vi "Process Image.vi"(4 "Path Angle":dbl, 6 "Camera Angle":dbl, 7 "?":T1, 8 "Error In":errorcluster, 9 "FOV":dbl[](array[numeric]), 10 "Process Memory":T2, 11 "Acquired Image":T2) -> (0 "Error Out":errorcluster, 1 "Particle Locations":dbl[][](array[numeric]) format="%.2f", 3 "Processed Image":T2)   [LabVIEW 2018]
uses:
  <vilib>/vision/Image Controls.llb/IMAQ Image.ctl
  <vilib>/vision/NI_Vision_Development_Module.lvlib
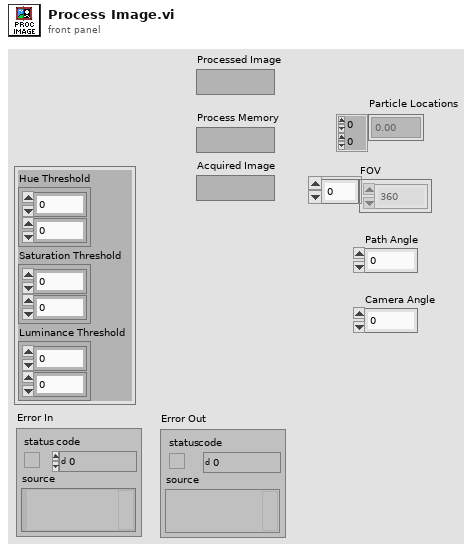
[diagram p1: front panel]
types:
  T1 = cluster{"Hue Threshold":cluster{i32, i32}, "Saturation Threshold":cluster{i32, i32}, "Luminance Threshold":cluster{i32, i32}}
  T2 = typedef "IMAQ Image.ctl" = refnum<image>
  T3 = cluster{"Blue or Luma":u8, "Green or Sat Plane":u8, "Red or Hue Plane":u8, "Alpha":u8}
  T4 = typedef "IMAQ Circle" = cluster{"Center X":i32, "Center Y":i32, "Inner Radius":i32, "Outer Radius":i32, "Start Angle":dbl, "End Angle":dbl}
  T5 = typedef "Particle Parameters" = i32
  T6 = typedef "ROI Descriptor" = cluster{"Global Rectangle":i32[], "Contours":cluster{"ID":enum32{"External", "Internal"}, "Type":u32, "Coordinates":i32[]}[]}
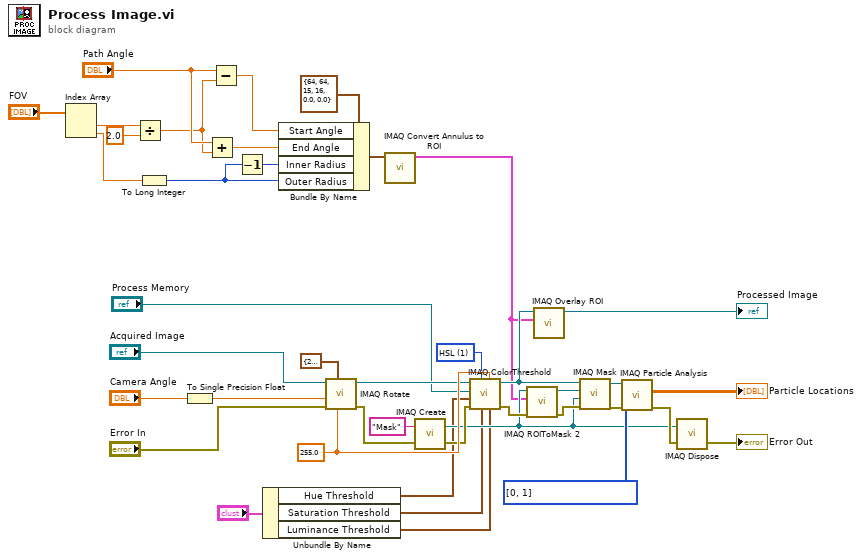
[diagram p0: block diagram]
diagram:
  w2 = u16 1 items=["RGB", "HSL", "HSV", "HSI"] ("Color Mode")
  w34 = T5[] [0, 1] items=["Center of Mass X", "Center of Mass Y", "First Pixel X", "First Pixel Y", "Bounding Rect Left", "Bounding Rect Top", "Bounding Rect Right", "Bounding Rect Bottom", "Max Feret Diameter Start X", "Max Feret Diameter Start Y", "Max Feret Diameter End X", "Max Feret Diameter End Y", "Max Horiz. Segment Length Left", "Max Horiz. Segment Length Right", "Max Horiz. Segment Length Row", "-", "Bounding Rect Width", "Bounding Rect Height", "Bounding Rect Diagonal", "Perimeter", "Convex Hull Perimeter", "Holes' Perimeter", "Max Feret Diameter", "Equivalent Ellipse Major Axis", "Equivalent Ellipse Minor Axis", "Equivalent Ellipse Minor Axis (Feret)", "Equivalent Rect Long Side", "Equivalent Rect Short Side", "Equivalent Rect Diagonal", "Equivalent Rect Short Side (Feret)", "Average Horiz. Segment Length", "Average Vert. Segment Length", "Hydraulic Radius", "Waddel Disk Diameter", "-", "Area", "Holes' Area", "Particle & Holes' Area", "Convex Hull Area", "Image Area", "-", "Number of Holes", "Number of Horiz. Segments", "Number of Vert. Segments", "-", "Orientation", "Max Feret Diameter Orientation", "-", "% Area/Image Area", "% Area/(Particle & Holes' Area)", "Ratio of Equivalent Ellipse Axes", "Ratio of Equivalent Rect Sides", "-", "Elongation Factor", "Compactness Factor", "Heywood Circularity Factor", "Type Factor", "-", "Sum X", "Sum Y", "Sum XX", "Sum XY", "Sum YY", "Sum XXX", "Sum XXY", "Sum XYY", "Sum YYY", "-", "Moment of Inertia XX", "Moment of Inertia XY", "Moment of Inertia YY", "Moment of Inertia XXX", "Moment of Inertia XXY", "Moment of Inertia XYY", "Moment of Inertia YYY", "Norm. Moment of Inertia XX", "Norm. Moment of Inertia XY", "Norm. Moment of Inertia YY", "Norm. Moment of Inertia XXX", "Norm. Moment of Inertia XXY", "Norm. Moment of Inertia XYY", "Norm. Moment of Inertia YYY", "Hu Moment 1", "Hu Moment 2", "Hu Moment 3", "Hu Moment 4", "Hu Moment 5", "Hu Moment 6", "Hu Moment 7"] ("Pixel Measurements")
  w41 = sgl 255.0 ("Replace Value")
  n1 = Index Array(array="FOV") -> (element #1=w10:dbl, element #2=w9:dbl)  [unwired: 2 in]
  n2 = Divide(x=w10, y=2.0) -> (x/y=w14:dbl)
  n3 = To Long Integer(number=w9) -> (32bit integer=w8:i32)
  n4 = To Single Precision Float(number="Camera Angle") -> (single precision float=w40:sgl)
  n5 = Add(x="Path Angle", y=w14) -> (x+y=w13:dbl)
  n6 = Subtract(x="Path Angle", y=w14) -> (x-y=w12:dbl)
  n7 = Decrement(x=w8) -> (x-1=w7:i32)
  n8 = Unbundle By Name("?") -> ("Hue Threshold"=w5:cluster{i32, i32}, "Saturation Threshold"=w4:cluster{i32, i32}, "Luminance Threshold"=w3:cluster{i32, i32})
  n9 = Bundle By Name(cluster=T4 {"Center X"=64, "Center Y"=64, "Inner Radius"=15, "Outer Radius"=16, "Start Angle"=0.0, "End Angle"=0.0} ("Annulus"), "Start Angle"=w12, "End Angle"=w13, "Inner Radius"=w7, "Outer Radius"=w8) -> (w18:T4)
  n10 = call "IMAQ Rotate"("Replace Value"=w41, "Color Replace Value"=T3 {"Blue or Luma"=255, "Green or Sat Plane"=255, "Red or Hue Plane"=255, "Alpha"=255}, "error in (no error)"="Error In", "Angle (degrees)"=w40, "Image Src"="Acquired Image") -> ("error out"=w24:errorcluster, "Image Dst Out"=w29:T2)  [unwired: 5 in]
  n11 = call "IMAQ Convert Annulus to ROI"("Annulus"=w18) -> ("ROI Descriptor"=w17:T6)  [unwired: 8 in, 1 out]
  n12 = call "IMAQ Create"("Image Name"="Mask", "error in (no error)"=w24) -> ("New Image"=w20:T2, "error out"=w23:errorcluster)  [unwired: 3 in]
  n13 = call "IMAQ ColorThreshold"("Blue or Luma or Val or Inten Range"=w3, "Replace Value"=w41, "Green or Sat Range"=w4, "Color Mode"=w2, "error in (no error)"=w23, "Red or Hue Range"=w5, "Image Dst"="Process Memory", "Image Src"=w29) -> ("error out"=w38:errorcluster, "Image Dst Out"=w27:T2)  [unwired: 2 in]
  n14 = call "IMAQ ROIToMask 2"("error in (no error)"=w38, "ROI Descriptor"=w17, "Image"=w20) -> ("error out"=w39:errorcluster, "Image Out"=w37:T2)  [unwired: 6 in, 1 out]
  n15 = call "IMAQ Overlay ROI"("ROI Descriptor"=w17, "Image"=w27) -> ("Image Out"=→"Processed Image":T2)  [unwired: 8 in, 1 out]
  n16 = call "IMAQ Mask"("error in (no error)"=w39, "Image Dst"=w20, "Image Mask"=w37, "Image Src"=w27) -> ("error out"=w36:errorcluster, "Image Dst Out"=w35:T2)  [unwired: 1 in]
  n17 = call "IMAQ Particle Analysis"("error in (no error)"=w36, "Pixel Measurements"=w34, "Image"=w35) -> ("error out"=w22:errorcluster, "Particle Measurements (Pixels)"=→"Particle Locations":dbl[][])  [unwired: 3 in, 4 out]
  n18 = call "IMAQ Dispose"("Image"=w20, "error in (no error)"=w22) -> ("error out"=→"Error Out":errorcluster)  [unwired: 4 in]
